vi "System Ready.vi"(8 "error in":errorcluster, 11 "CPC in":refnum<class "CPC.lvclass">) -> (0 "error out":errorcluster, 2 "Ready?":bool, 3 "CPC out":refnum<class "CPC.lvclass">)   [LabVIEW 2014, in "CPC.lvclass"]
doc: "Read environment. READY implies that the temperatures, flow and alcohol level are all within the operating range. Values are:\n* READY\n* NOTREADY"
uses:
  CPC.lvclass
  Controls/3022A/Enum Cmd.ctl
  3022A/3022A.lvclass
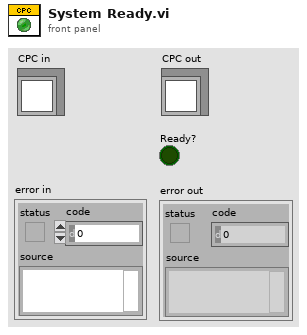
[diagram p1: front panel]
types:
  T1 = typedef "3022A.lvclass/Enum Cmd.ctl" = enum8{"CALIBRATE", "GET CAL DATA", "DUMP", "ESCAPE", "ID CAL LABEL", "INPUT CAL LABEL", "LIQUID LEVEL", "CONDENSER T", "SATURATOR T", "OPTICS T", "GET FLOW RATE", "READ ENV", "READ REF DETECTOR", "READ DETECTOR V", "READ 200 s BUFFER", "READ 20 s BUFFER", "READ 2 s BUFFER", "READ 1 s BUFFER", "READ PHOTOMETRIC CONC", "READ FP CONC", "READ MICROPROCESSOR PUMP CTL", "SENSOR", "SET VOLTAGE", "WRITE DISP MSG", "LASER OFF", "LASER ON", "PUMP OFF", "PUMP ON", "DRAIN", "FILL", "RESET CONC BUFFERS", "LOW FLOW MODE", "HIGH FLOW MODE"}
  T2 = cluster{"Cmd":T1, "x":i64, "y":i64, "Display":string}
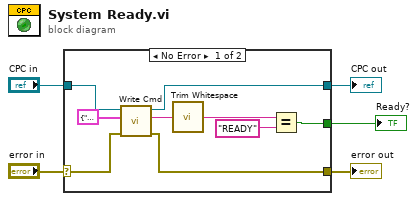
[diagram p0: block diagram]
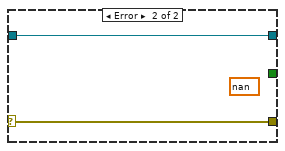
[diagram p2: hidden frame]
diagram:
  n1 = case shown="No Error" "error in" {
    selector: "error in" -> [w14 w16]
    tunnel: [w13 w16] -> w4
    tunnel: [w11 w15] -> w2
    tunnel: "CPC in" -> [w12 w15]
    tunnel: [w8 _] -> w1
    frame No Error {
      n2 = call-dynamic "Write Cmd.vi"("error in"=w14, "CmdStruct"=T2 {"Cmd"=enum."READ ENV", "x"=0, "y"=0, "Display"=""}, "CPC in"=w12) -> ("error out"=w13:errorcluster, "Buffer"=w7:string, "CPC out"=w11:refnum<class "CPC.lvclass">)  [unwired: 6 in]
      n3 = call <vilib>:"Trim Whitespace.vi"("string"=w7) -> ("trimmed string"=w6:string)  [unwired: 1 in]
      n4 = Equal?(x=w6, y="READY") -> (x = y?=w8:bool)
    }
    frame Error {
      (unwired) nan
    }
  }
  "error out" <- w4
  "CPC out" <- w2
  "Ready?" <- w1
